vi "Configure Input Output Amplitude Sweep.vi"(6 "Enable Log (F: Disabled)":bool, 7 "Stop Amplitude (0 Vrms)":dbl, 8 "error in (no error)":errorcluster, 9 "Number Of Steps (0)":i32, 10 "Start Amplitude (0 Vrms)":dbl, 11 "VISA resource name":refnum<visa-resource-name>) -> (0 "error out":errorcluster, 3 "VISA resource name out":refnum<visa-resource-name>)   [LabVIEW 2014, in "Stanford Research SR1.lvlib"]
doc: "Configures the attributes for the Input Output Amplitude Sweep."
uses:
  Stanford Research SR1.lvlib
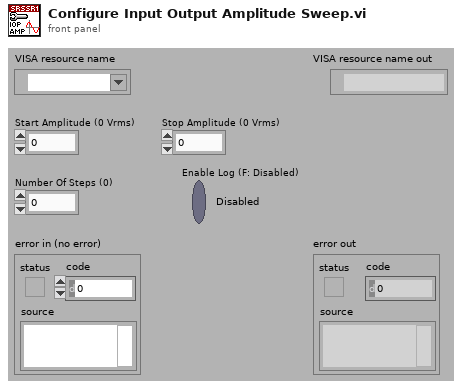
[diagram p1: front panel]
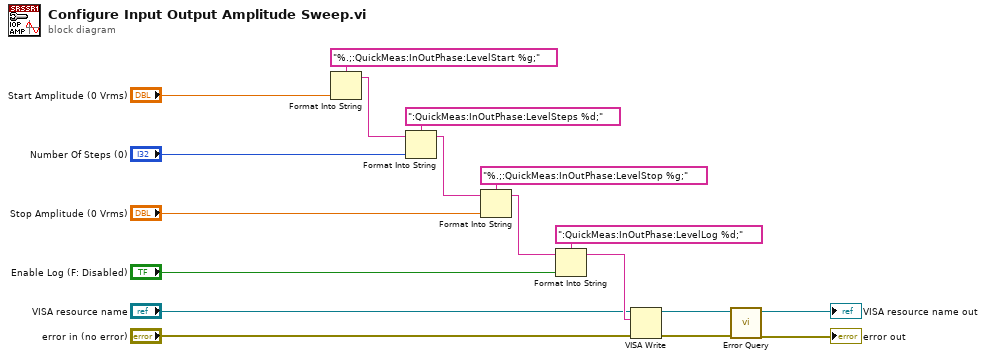
[diagram p0: block diagram]
diagram:
  n1 = Format Into String(format string="%.;:QuickMeas:InOutPhase:LevelStart %g;", "Start Amplitude (0 Vrms)") -> (resulting string=w16:string)  [unwired: 2 in, 1 out]
  n2 = Format Into String(format string=":QuickMeas:InOutPhase:LevelSteps %d;", initial string=w16, "Number Of Steps (0)") -> (resulting string=w13:string)  [unwired: 1 in, 1 out]
  n3 = Format Into String(format string="%.;:QuickMeas:InOutPhase:LevelStop %g;", initial string=w13, "Stop Amplitude (0 Vrms)") -> (resulting string=w10:string)  [unwired: 1 in, 1 out]
  n4 = Format Into String(format string=":QuickMeas:InOutPhase:LevelLog %d;", initial string=w10, "Enable Log (F: Disabled)") -> (resulting string=w7:string)  [unwired: 1 in, 1 out]
  n5 = VISA Write(VISA resource name="VISA resource name", write buffer=w7, error in (no error)="error in (no error)") -> (VISA resource name out=w4:refnum<visa-resource-name>, error out=w3:errorcluster)  [unwired: 1 out]
  n6 = call "Error Query.vi"("error in (no error)"=w3, "VISA resource name"=w4) -> ("error out"=→"error out":errorcluster, "VISA resource name out"=→"VISA resource name out":refnum<visa-resource-name>)  [unwired: 6 in, 2 out]
